vi "z keyexpr as view string.vi"(8 "error in (no error)":errorcluster, 10 "out_string":cluster{}, 11 "this_":cluster{}) -> (0 "error out":errorcluster, 2 "out_string out":cluster{})   [LabVIEW 2021, in "zenohc.lvlib"]
doc: "void z_keyexpr_as_view_string(const struct z_loaned_keyexpr_t *this_,\n struct z_view_string_t *out_string);"
uses:
  zenohc.lvlib
  zenohc.dll
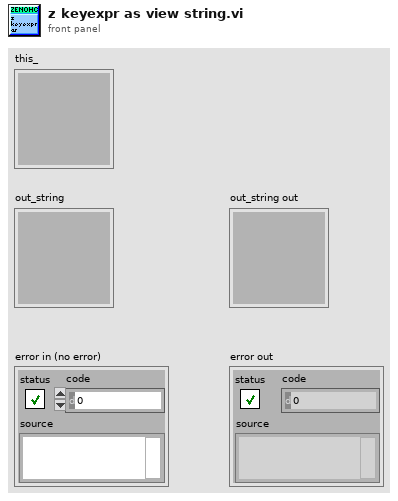
[diagram p1: front panel]
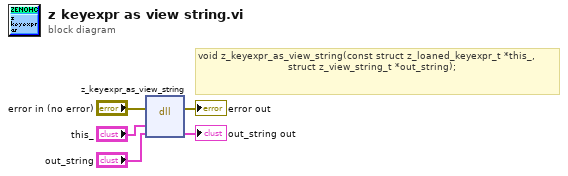
[diagram p0: block diagram]
diagram:
  # "void z_keyexpr_as_view_string(const struct z_loaned_keyexpr_t *this_,\n                              struct z_view_string_t *out_string);"
  n1 = dll-call lib="D:/dev/zenoh_labview/zenohc/zenohc.*" fn="z_keyexpr_as_view_string"(error in="error in (no error)", "this_"="this_", "out_string"="out_string") -> (error out=→"error out":errorcluster, "out_string"=→"out_string out":cluster{})  [unwired: 4 in, 1 out]
